vi "kalman_filter.vi"(0 "measured value":dbl, 12 "q":dbl=50.0, 13 "r":dbl=0.1) -> (4 "x_out":dbl, 8 "p_out":dbl, 15 "k_out":dbl)   [LabVIEW 2012]
panel:
  # "q = process noise covariance\nr = measurement noise covariance"
  # "r > 1\nq < 1"
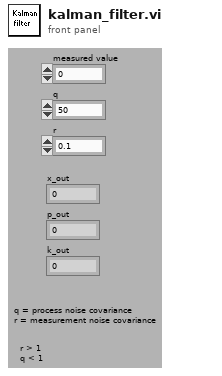
[diagram p1: front panel]
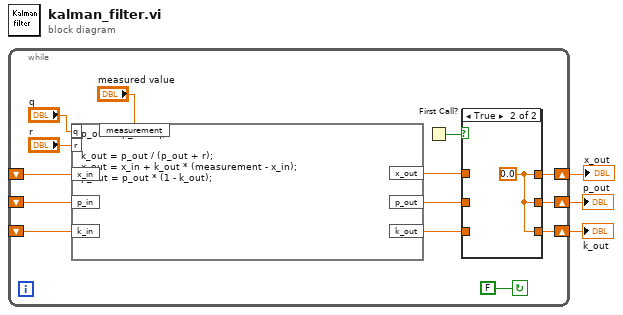
[diagram p0: block diagram]
diagram:
  n1 = while {
    shift-right: [w8] -> w2
    shift-left: _ -> [w12]
    shift-right: [w9] -> w3
    shift-left: _ -> [w13]
    shift-right: [w7] -> w1
    shift-left: _ -> [w11]
    stop <- FALSE continue-if-true
    n2 = formula code="p_out = p_in + q;\n\nk_out = p_out / (p_out + r);\nx_out = x_in + k_out * (measurement - x_in);\np_out = p_out * (1 - k_out);"("x_in"=w13, "p_in"=w12, "k_in"=w11, "q"="q", "measurement"="measured value", "r"="r") -> ("x_out"=w6:dbl, "p_out"=w5:dbl, "k_out"=w4:dbl)
    n3 = First Call?() -> (First Call?: T/F=w10:bool)
    n4 = case shown="True" w10 {
      tunnel: [w20 w21] -> w9
      tunnel: [w19 w21] -> w8
      tunnel: [w18 w21] -> w7
      tunnel: w6 -> [w20 _]
      tunnel: w5 -> [w19 _]
      tunnel: w4 -> [w18 _]
      frame False {
      }
      frame True {
        w21 = 0.0
      }
    }
  }
  "x_out" <- w3
  "p_out" <- w2
  "k_out" <- w1
